vi "FindMaxCountsinTrace_sub.vi"(0 "Macros":i32[](array[numeric]), 1 "bin time (ns)":i32=10000) -> (2 "Output":bool, 3 "tracelength":i32, 4 "max counts":i32)   [LabVIEW 2009]
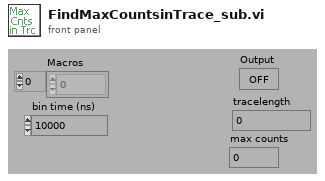
[diagram p1: front panel]
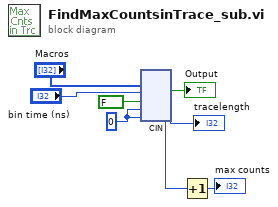
[diagram p0: block diagram]
diagram:
  w5 = 0
  n1 = cin("Macros", "bin time (ns)", FALSE, w5, w5) -> (→"Output":bool, →"tracelength":i32, w2:i32)  [unwired: 2 in]
  n2 = Increment(x=w2) -> (x+1=→"max counts":i32)
